vi "Protected Signal.vi"(8 "error in (no error)":errorcluster, 11 "Node Ptr":T1 format="%.0x") -> (0 "error out":errorcluster)   [LabVIEW 2015, in "Diagnostics Addon System Explorer.lvlib"]
uses:
  Diagnostics Addon System Explorer.lvlib
  <vilib>/NI Veristand/Custom Device API/Custom Device Item Ref.ctl
  <vilib>/NI Veristand/Custom Device API/Custom Device API.lvlib
panel:
  in  "Header":cluster{"Section Name":string}={"Section Name"="Custom Device Item Settings"}
  out "Name":string
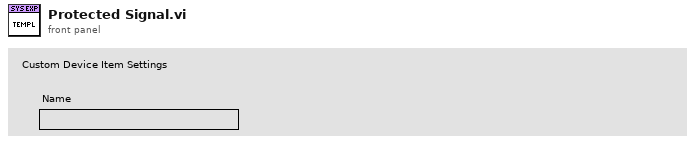
[diagram p1: front panel]
types:
  T1 = typedef "Custom Device API.lvlib/Custom Device Item Ref.ctl" = u64
  T2 = typedef "Custom Device API.lvlib/Custom Device Item Info.ctl" = cluster{"Name":string, "Is Channel":bool, "GUID":string, "Is Waveform":bool}
  T3 = typedef "Custom Device API.lvlib/Custom Device Commands.ctl" = enum16{"Default", "Item renamed", "Shutdown", "Dynamic button pressed"}
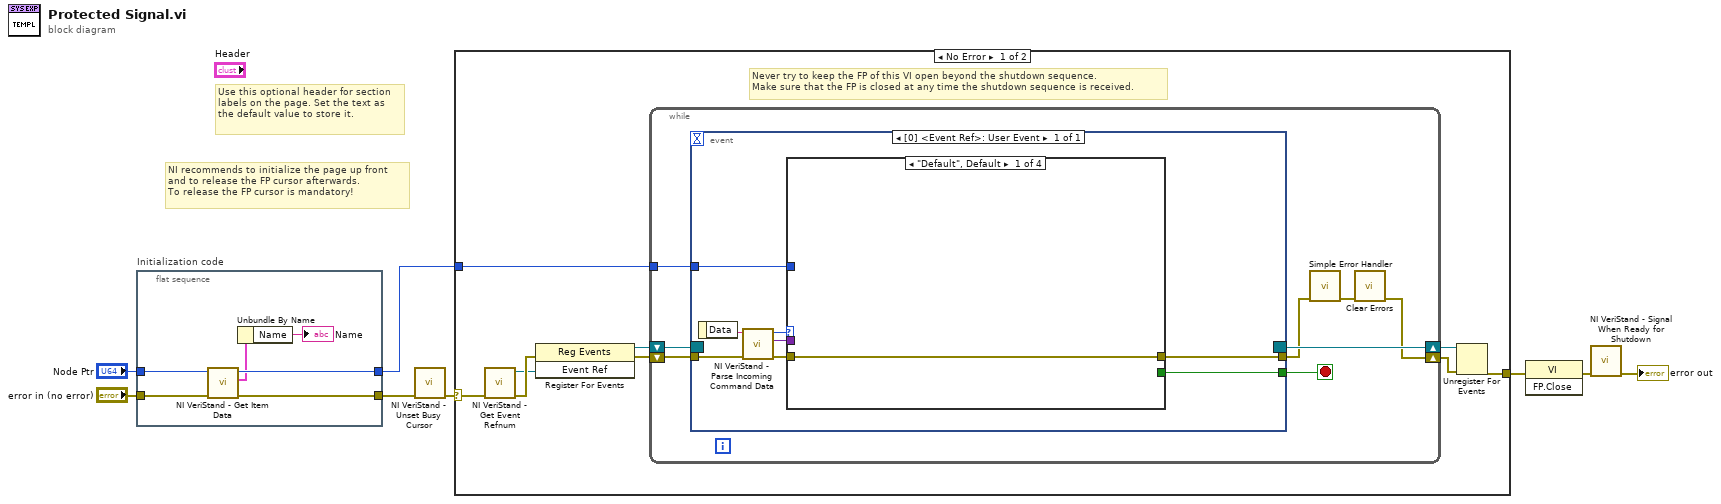
[diagram p0: block diagram]
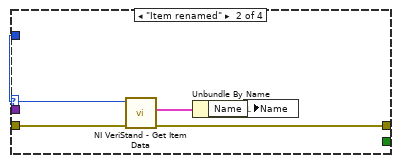
[diagram p2: hidden frame]
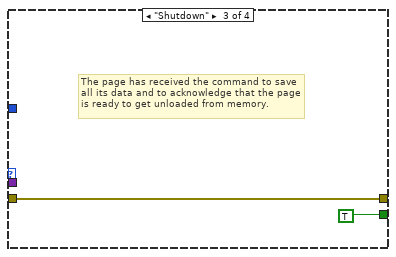
[diagram p3: hidden frame]
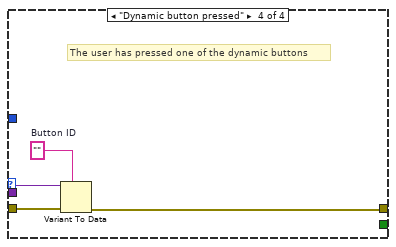
[diagram p4: hidden frame]
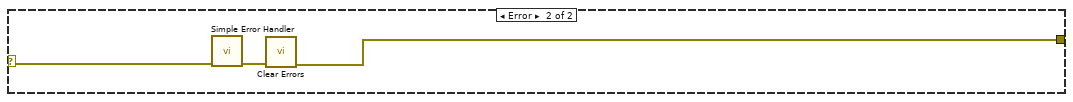
[diagram p5: hidden frame]
diagram:
  # "Use this optional header for section labels on the page. Set the text as the default value to store it."
  # "NI recommends to initialize the page up front\nand to release the FP cursor afterwards.\nTo release the FP cursor is mandatory!"
  n1 = flat-sequence "Initialization code" {
    tunnel: "error in (no error)" -> [w10]
    tunnel: "Node Ptr" -> [w9]
    tunnel: [w12] -> w4
    tunnel: [w14] -> w1
    frame #0 {
      n2 = call <vilib>:"NI VeriStand - Get Item Data.vi"("error in (no error)"=w10, "Item Ref in"=w9) -> ("error out"=w12:errorcluster, "Item Info"=w13:T2, "Item Ref out"=w14:T1)  [unwired: 7 out]
      n3 = Unbundle By Name(w13) -> ("Name"=→"Name":string)
    }
  }
  n4 = call <vilib>:"NI VeriStand - Unset Busy Cursor.vi"("error in (no error)"=w4) -> ("error out"=w3:errorcluster)  [unwired: 10 out]
  n5 = case shown="No Error" w3 {
    selector: w3 -> [w15 w54]
    tunnel: [w20 w52] -> w8
    tunnel: w1 -> [w16 _]
    frame No Error {
      # "Never try to keep the FP of this VI open beyond the shutdown sequence.\nMake sure that the FP is closed at any time the shutdown sequence is received."
      n6 = call <vilib>:"NI VeriStand - Get Event Refnum.vi"("error in (no error)"=w15) -> ("error out"=w23:errorcluster, "Event Ref"=w19:refnum<user-event>)  [unwired: 9 out]
      n7 = register-events(error in=w23, w19) -> (reference out=w17:refnum<event-registration>, error out=w18:errorcluster)  [unwired: 1 in]
      n8 = while {
        tunnel: w16 -> [w27]
        shift-right: [w24] -> w21
        shift-left: w18 -> [w30]
        shift-right: [w31] -> w22
        shift-left: w17 -> [w29]
        stop <- w28 stop-if-true
        n9 = event shown="[0] <Event Ref>: User Event" {
          selector: w29 -> [_]
          dyn-events: [_] -> w31
          timeout: _ -> [_]
          tunnel: w30 -> [w39]
          tunnel: [w35] -> w28
          tunnel: [w34] -> w26
          tunnel: w27 -> [w33]
          event User Event {
            n10 = event-data() -> ("Data"=w38:string)  [unwired: 1 out]
            n11 = call <vilib>:"NI VeriStand - Parse Incoming Command Data.vi"("error in (no error)"=w39, "Incoming data"=w38) -> ("error out"=w37:errorcluster, "Outgoing data"=w32:variant, "Action"=w36:T3)  [unwired: 7 out]
            n12 = case shown="\"Default\", Default" w36 {
              tunnel: w37 -> [w40 w45 w46 w51]
              tunnel: [_ _ TRUE _] -> w35
              tunnel: [w40 w42 w46 w48] -> w34
              tunnel: w33 -> [_ w44 _ _]
              tunnel: w32 -> [_ _ _ w50]
              frame "Default", Default {
              }
              frame "Item renamed" {
                n13 = call <vilib>:"NI VeriStand - Get Item Data.vi"("error in (no error)"=w45, "Item Ref in"=w44) -> ("error out"=w42:errorcluster, "Item Info"=w43:T2)  [unwired: 8 out]
                n14 = Unbundle By Name(w43) -> ("Name"=w41:string)
                n15 = local write "Name"(w41) -> ()
              }
              frame "Shutdown" {
                # "The page has received the command to save all its data and to acknowledge that the page is ready to get unloaded from memory."
              }
              frame "Dynamic button pressed" {
                w49 = ""  # Button ID
                # "The user has pressed one of the dynamic buttons"
                n16 = Variant To Data(error in=w51, type=w49, Variant=w50) -> (error out=w48:errorcluster)  [unwired: 1 out]
              }
            }
          }
        }
        n17 = call <vilib>:"Simple Error Handler.vi"("error in (no error)"=w26) -> ("error out"=w25:errorcluster)  [unwired: 1 in, 7 out]
        n18 = call <vilib>:"Clear Errors.vi"("error in (no error)"=w25) -> ("error out"=w24:errorcluster)  [unwired: 1 in, 5 out]
      }
      n19 = Unregister For Events(event registration refnum=w22, error in=w21) -> (error out=w20:errorcluster)
    }
    frame Error {
      n20 = call <vilib>:"Simple Error Handler.vi"("error in (no error)"=w54) -> ("error out"=w53:errorcluster)  [unwired: 1 in, 7 out]
      n21 = call <vilib>:"Clear Errors.vi"("error in (no error)"=w53) -> ("error out"=w52:errorcluster)  [unwired: 1 in, 5 out]
    }
  }
  n22 = invoke class="VI" method="FP.Close"(error in=w8) -> (error out=w7:errorcluster)  [unwired: 2 in, 2 out]
  n23 = call <vilib>:"NI VeriStand - Signal When Ready for Shutdown.vi"("error in (no error)"=w7) -> ("error out"=→"error out":errorcluster)  [unwired: 10 out]
